vi "Add Res Card.vi"(8 "error in (no error)":errorcluster, 11 "Node Ptr":u64 format="%.0x") -> (0 "error out":errorcluster)   [LabVIEW 2014, in "SLSC configuration System Explorer.lvlib"]
uses:
  SLSC configuration System Explorer.lvlib
  <vilib>/NI Veristand/Custom Device API/Custom Device Channel.ctl
  <vilib>/NI Veristand/Custom Device API/Custom Device Channel Type.ctl
  Shared/Constants.vi
  <vilib>/NI Veristand/Custom Device API/Set Item Property (Variant).vi
  <vilib>/NI Veristand/Custom Device API/Set Item Property (U16).vi
  Shared/SLSC configuration Shared.lvlib
  <vilib>/NI Veristand/Custom Device API/Custom Device API.lvlib
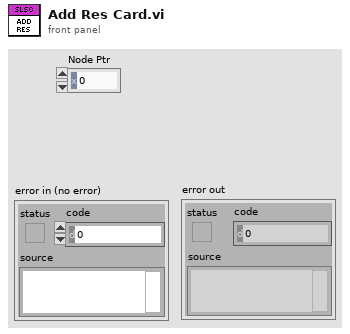
[diagram p1: front panel]
types:
  T1 = typedef "SLSC configuration Shared.lvlib/Card Postion.ctl" = cluster{"Chassis #":u8, "Slot #":u8}
  T2 = typedef "Custom Device API.lvlib/Custom Device Item Ref.ctl" = u64
  T3 = typedef "Custom Device API.lvlib/Custom Device Channel Type.ctl" = enum16{"Input", "Output"}
  T4 = typedef "Custom Device API.lvlib/Custom Device Channel.ctl" = cluster{"Type":T3, "Units":string, "Default Value":dbl, "Faultable":bool, "Scalable":bool}
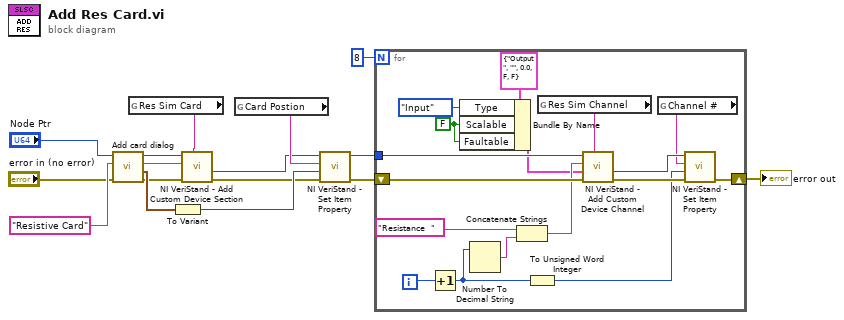
[diagram p0: block diagram]
diagram:
  n1 = call "Add card dialog.vi"("error in (no error)"="error in (no error)", "Card Type in"="Resistive Card" ("Section Name"), "Node Ptr"="Node Ptr") -> ("error out"=w8:errorcluster, "Card position out"=w12:T1, "Name out"=w9:string, "Node Ptr out"=w10:u64)  [unwired: 4 in, 1 out]
  n2 = global read "Constants.vi" "Res Sim Card"() -> (w7:string)
  n3 = To Variant(anything=w12) -> (Variant=w13:variant)
  n4 = call <vilib>:"NI VeriStand - Add Custom Device Section.vi"("GUID (Default Section)"=w7, "error in (no error)"=w8, "Section Name"=w9, "Parent Ref in"=w10) -> ("error out"=w6:errorcluster, "Section Ptr"=w11:T2)  [unwired: 4 in, 2 out]
  n5 = global read "Constants.vi" "Card Postion"() -> (w14:string)
  n6 = call-poly <vilib>:"NI VeriStand - Set Item Property.vi"("error in (no error)"=w6, "Value"=w13, "Property Name"=w14, "Item Ref in"=w11) -> ("error out"=w4:errorcluster, "Item Ref out"=w3:T2)  [unwired: 5 in, 1 out]
  n7 = for {
    N: 8 -> [_]
    shift-right: [w25] -> w15
    shift-left: w4 -> [w31]
    tunnel: w3 -> [w32]
    i -> [w33]
    w17 = FALSE ("Scalable")
    n8 = Increment(x=w33) -> (x+1=w22:i32)
    n9 = Bundle By Name(cluster=T4 {"Type"=enum."Output", "Units"="", "Default Value"=0.0, "Faultable"=FALSE, "Scalable"=FALSE} ("Channel"), "Type"=Custom_Device_Channel_Type."Input", "Scalable"=w17, "Faultable"=w17) -> (w19:T4)
    n10 = Number To Decimal String(number=w22) -> (decimal integer string=w29:string)  [unwired: 1 in]
    n11 = Concatenate Strings("Resistance  " ("Channel Name"), w29) -> (w27:string)
    n12 = To Unsigned Word Integer(number=w22) -> (unsigned 16bit integer=w21:u16)
    n13 = global read "Constants.vi" "Res Sim Channel"() -> (w30:string)
    n14 = call <vilib>:"NI VeriStand - Add Custom Device Channel.vi"("GUID (Default Channel)"=w30, "error in (no error)"=w31, "Channel"=w19, "Channel Name"=w27, "Parent Ref in"=w32) -> ("error out"=w26:errorcluster, "Channel Ref"=w24:T2)  [unwired: 3 in, 2 out]
    n15 = global read "Constants.vi" "Channel #"() -> (w23:string)
    n16 = call-poly <vilib>:"NI VeriStand - Set Item Property.vi"("error in (no error)"=w26, "Value"=w21, "Property Name"=w23, "Item Ref in"=w24) -> ("error out"=w25:errorcluster)  [unwired: 5 in, 2 out]
  }
  "error out" <- w15
